vi "SeCrTs-AI Cumulative Sequence Check.vi"(5 "output cluster":T1, 8 "AI DATA":dbl, 9 "CDT":dbl, 10 "Loop no":i32) -> (1 "Failure case Seq":string, 2 "Boolean":bool, 3 "String":string)   [LabVIEW 2022 SP3]
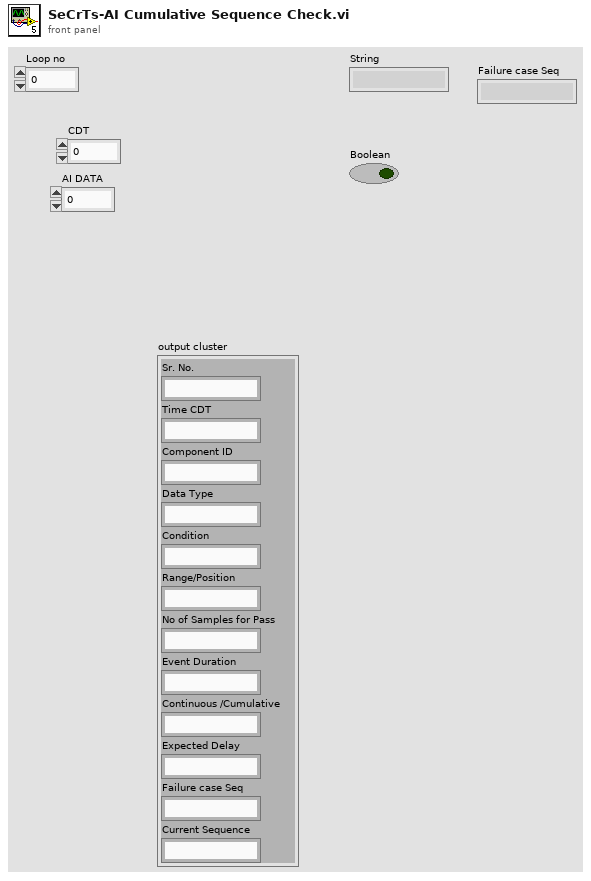
[diagram p1: front panel]
types:
  T1 = cluster{"Sr. No.":string, "Time CDT":string, "Component ID":string, "Data Type":string, "Condition":string, "Range/Position":string, "No of Samples for Pass":string, "Event Duration":string, "Continuous /Cumulative":string, "Expected Delay":string, "Failure case Seq":string, "Current Sequence":string}
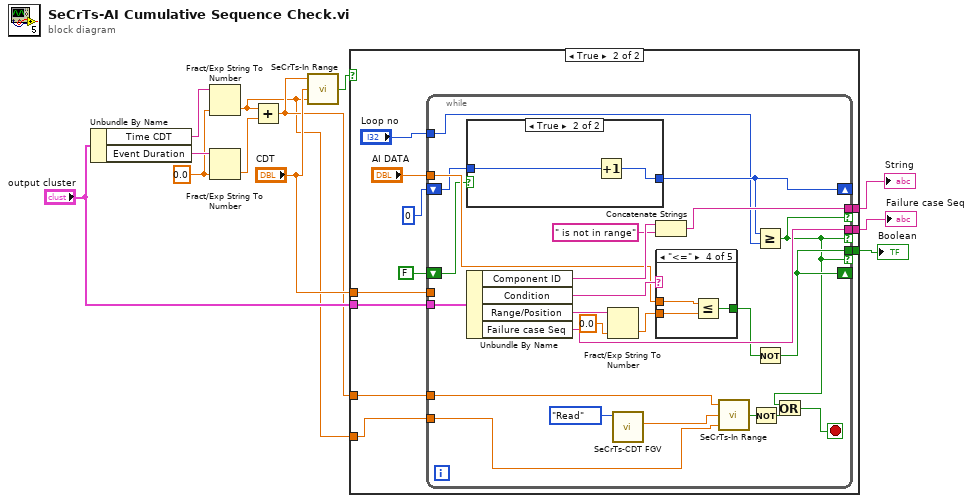
[diagram p0: block diagram]
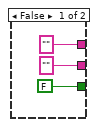
[diagram p2: hidden frame]
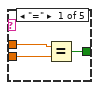
[diagram p3: hidden frame]
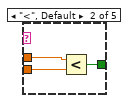
[diagram p4: hidden frame]
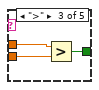
[diagram p5: hidden frame]
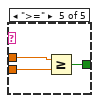
[diagram p6: hidden frame]
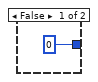
[diagram p7: hidden frame]
diagram:
  w8 = 0.0
  n1 = Unbundle By Name("output cluster") -> ("Time CDT"=w10:string, "Event Duration"=w9:string)
  n2 = Fract/Exp String To Number(string=w10, default (0 dbl)=w8) -> (number=w1:dbl)  [unwired: 2 in, 1 out]
  n3 = Fract/Exp String To Number(string=w9, default (0 dbl)=w8) -> (number=w11:dbl)  [unwired: 2 in, 1 out]
  n4 = Add(x=w1, y=w11) -> (x+y=w2:dbl)
  n5 = call "SeCrTs-In Range.vi"("Min"=w1, "X"="CDT", "Max"=w2) -> ("In Range"=w7:bool)  [unwired: 2 in]
  n6 = case shown="True" w7 {
    tunnel: "output cluster" -> [_ w24]
    tunnel: "CDT" -> [_ w23]
    tunnel: [FALSE w22] -> w6
    tunnel: ["" w21] -> w5
    tunnel: ["" ("Failure case Seq") w20] -> w4
    tunnel: w2 -> [_ w17]
    tunnel: w1 -> [_ w16]
    frame False {
    }
    frame True {
      n7 = while {
        tunnel: w24 -> [w50]
        tunnel: [w46] -> w21 if=w29
        shift-right: [w40] -> _
        shift-left: FALSE -> [w43]
        tunnel: "AI DATA" -> [w45]
        shift-right: [w42] -> _
        shift-left: 0 ("Numeric") -> [w44]
        tunnel: [w41] -> w20 if=w29
        tunnel: [w40] -> w22 if=w29
        tunnel: w23 -> [_]
        tunnel: "Loop no" -> [w35]
        tunnel: w17 -> [w28]
        tunnel: w16 -> [w27]
        stop <- w30 stop-if-true
        n8 = case shown="True" w43 {
          tunnel: [0 w68] -> w42
          tunnel: w44 -> [_ w67]
          frame False {
          }
          frame True {
            n9 = Increment(x=w67) -> (x+1=w68:i32)
          }
        }
        n10 = Unbundle By Name(w50) -> ("Component ID"=w47:string, "Condition"=w48:string, "Range/Position"=w49:string, "Failure case Seq"=w41:string)
        n11 = Fract/Exp String To Number(string=w49, default (0 dbl)=0.0) -> (number=w38:dbl)  [unwired: 2 in, 1 out]
        n12 = call "SeCrTs-CDT FGV.vi"("Write/Read"=enum16{"Write", "Read"}."Read") -> ("CDT Out"=w33:dbl)  [unwired: 9 in, 1 out]
        n13 = Concatenate Strings(w47, " is not in range" ("string")) -> (w46:string)
        n14 = case shown="\"<=\"" w48 {
          tunnel: w38 -> [w53 w55 w58 w61 w64]
          tunnel: w45 -> [w52 w56 w59 w62 w65]
          tunnel: [w51 w54 w57 w60 w63] -> w36
          frame "=" {
            n15 = Equal?(x=w52, y=w53) -> (x = y?=w51:bool)
          }
          frame "<", Default {
            n16 = Less?(x=w56, y=w55) -> (x < y?=w54:bool)
          }
          frame ">" {
            n17 = Greater?(x=w59, y=w58) -> (0:w57:bool)
          }
          frame "<=" {
            n18 = Less Or Equal?(x=w62, y=w61) -> (x <= y?=w60:bool)
          }
          frame ">=" {
            n19 = Greater Or Equal?(x=w65, y=w64) -> (x >= y?=w63:bool)
          }
        }
        n20 = call "SeCrTs-In Range.vi"("Min"=w27, "X"=w33, "Max"=w28) -> ("In Range"=w31:bool)  [unwired: 2 in]
        n21 = Not(x=w31) -> (.not. x?=w32:bool)
        n22 = Greater Or Equal?(x=w42, y=w35) -> (x >= y?=w29:bool)
        n23 = Not(x=w36) -> (.not. x?=w40:bool)
        n24 = Or(x=w29, y=w32) -> (x .or. y?=w30:bool)
      }
    }
  }
  "Failure case Seq" <- w4
  "String" <- w5
  "Boolean" <- w6
